vi "ni_open.vi"(8 "error in":errorcluster) -> (0 "error out":errorcluster)   [LabVIEW 2011]
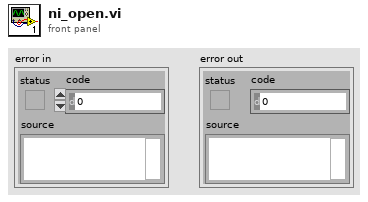
[diagram p1: front panel]
types:
  T1 = typedef "Board Id" = u8
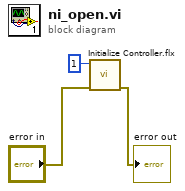
[diagram p0: block diagram]
diagram:
  n1 = call <vilib>:"Initialize Controller.flx"("error in (no error)"="error in", "Board ID"=T1 1) -> ("error out"=→"error out":errorcluster)  [unwired: 6 in, 1 out]
